vi "Apply Steering Angle.vi"(8 "error in (no error)":errorcluster, 10 "steering angle (rad)":dbl, 11 "steering wheel in":refnum<class "NI_Robotics_Steering Wheel.lvclass">) -> (0 "error out":errorcluster, 3 "steering wheel out":refnum<class "NI_Robotics_Steering Wheel.lvclass">)   [LabVIEW 2017, in "NI_Robotics_Steering Wheel.lvclass"]
uses:
  <vilib>/robotics/Steering/Steering Wheel/NI_Robotics_Steering Wheel.lvclass
  <vilib>/robotics/Steering/Steering Wheel/NI_Robotics_Steering Wheel.lvclass/NI_Robotics_Steering Wheel.ctl
  <vilib>/robotics/Actuation/Motor Communication/Check if Valid.vi
  <vilib>/robotics/Utilities/Generate Error.vi
  <vilib>/robotics/Actuation/Motor Communication/NI_Robotics_Motor Communication.lvclass
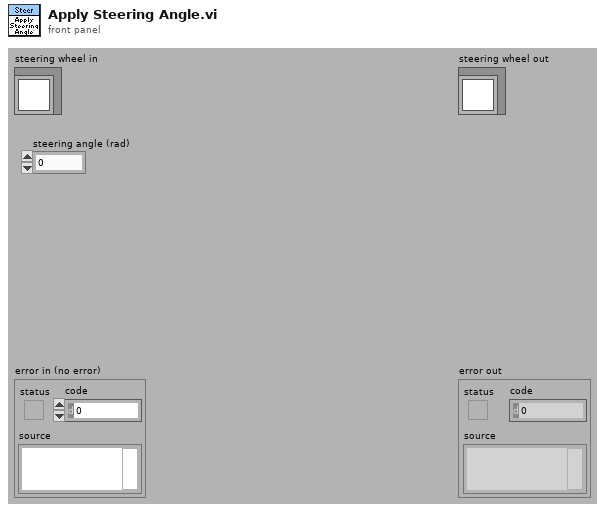
[diagram p1: front panel]
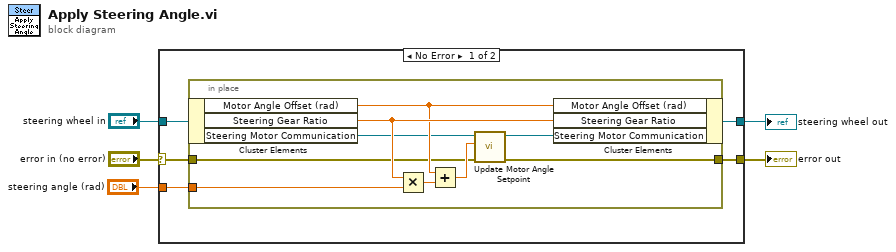
[diagram p0: block diagram]
diagram:
  n1 = case shown="No Error" "error in (no error)" {
    selector: "error in (no error)" -> [w9 w20]
    tunnel: "steering angle (rad)" -> [w7 _]
    tunnel: "steering wheel in" -> [w10 w21]
    tunnel: [w8 w21] -> w2
    tunnel: [w6 w20] -> w1
    frame No Error {
      n2 = in-place {
        in-place-border: w9 -> [w14]
        in-place-border: w7 -> [w18]
        in-place-border: [w13] -> w6
        n3 = in-place-cluster #1(w10) -> ("Motor Angle Offset (rad)"=w16:dbl, "Steering Gear Ratio"=w19:dbl, "Steering Motor Communication"=w12:refnum<class "NI_Robotics_Motor Communication.lvclass">)
        n4 = Multiply(x=w19, y=w18) -> (x*y=w17:dbl)
        n5 = Add(x=w16, y=w17) -> (x+y=w15:dbl)
        n6 = call <vilib>:"Update Motor Angle Setpoint.vi"("error in (no error)"=w14, "angle"=w15, "motor communication in"=w12) -> ("error out"=w13:errorcluster, "motor communication out"=w11:refnum<class "NI_Robotics_Motor Communication.lvclass">)  [unwired: 6 in, 1 out]
        n7 = in-place-cluster #1("Motor Angle Offset (rad)"=w16, "Steering Gear Ratio"=w19, "Steering Motor Communication"=w11) -> (w8:refnum<class "NI_Robotics_Steering Wheel.lvclass">)
      }
    }
    frame Error {
    }
  }
  "error out" <- w1
  "steering wheel out" <- w2
